vi "Launcher.vi"() -> ()   [LabVIEW 2024]
uses:
  Text/Text.lvclass
  C:/Users/burakkorkmaz/Desktop/Leveling/labview-design-patterns/Decorator Pattern/Labview/AbstractText/AbstractText.lvclass
  <vilib>/Utility/miscctls.llb/LVRectTypeDef.ctl
  BoldDecorator/BoldDecorator.lvclass
  ItalicDecorator/ItalicDecorator.lvclass
  UnderlineDecorator/UnderlineDecorator.lvclass
  AbstractText/AbstractText.lvclass
panel:
  out "Description":string
  out "Content":string
  in  "Add Underline":bool
  in  "Add Italic":bool
  in  "Add Bold":bool
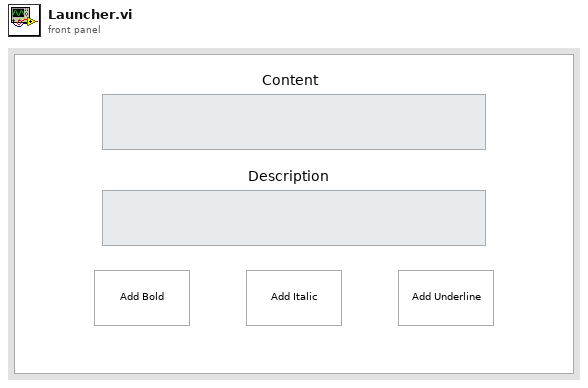
[diagram p1: front panel]
types:
  T1 = typedef "LVRectTypeDef.ctl" = cluster{"Left":i16, "Top":i16, "Right":i16, "Bottom":i16}
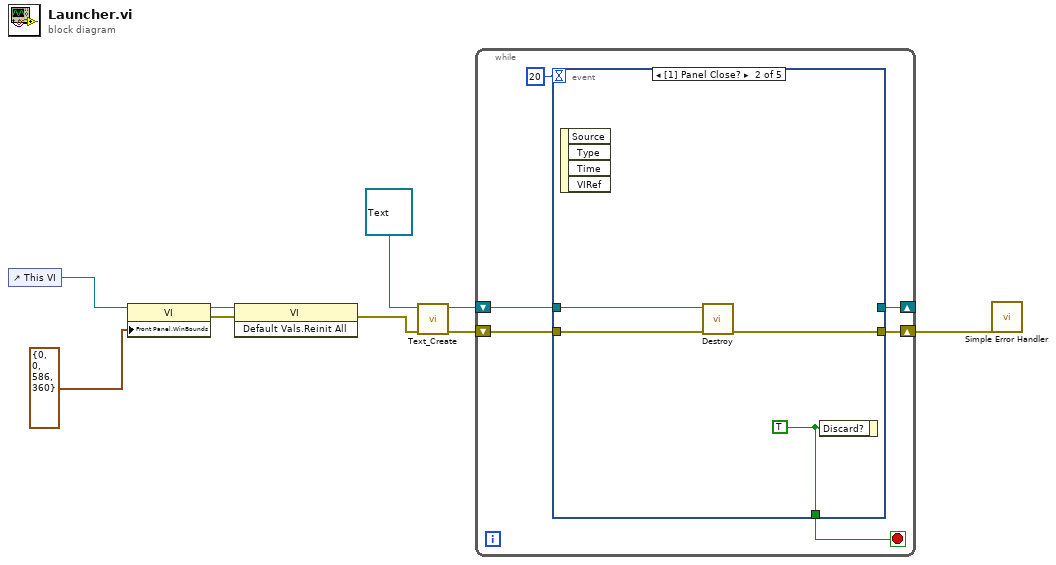
[diagram p0: block diagram]
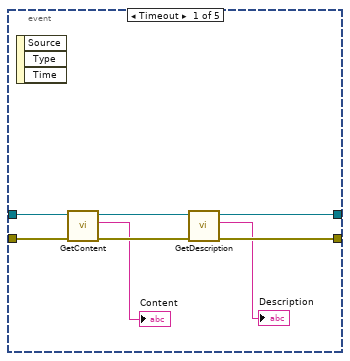
[diagram p2: hidden frame]
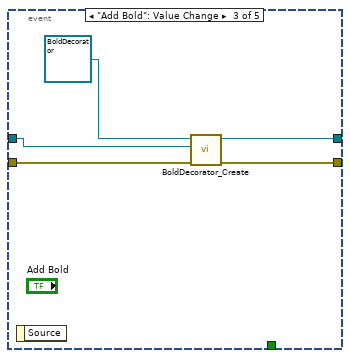
[diagram p3: hidden frame]
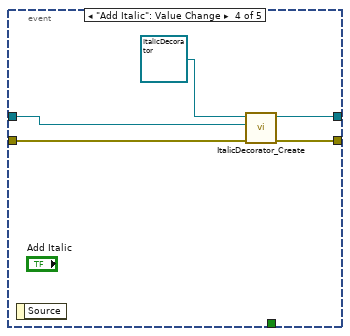
[diagram p4: hidden frame]
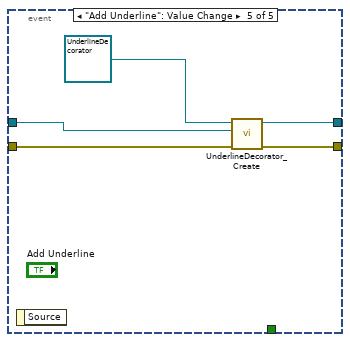
[diagram p5: hidden frame]
diagram:
  n1 = control-ref of="This VI"() -> (w9:refnum<vi>)
  n2 = property class="VI"(reference=w9, "Front Panel.WinBounds"=T1 {"Left"=0, "Top"=0, "Right"=586, "Bottom"=360} ("Front Panel Window:Window Bounds")) -> (reference out=w7:refnum<vi>, error out=w6:errorcluster)  [unwired: 1 in]
  n3 = invoke class="VI" method="Default Vals.Reinit All"(reference=w7, error in=w6) -> (error out=w5:errorcluster)  [unwired: 1 in, 2 out]
  n4 = call "Text_Create.vi"("Error In"=w5, "reference in"=refnum<class "Text.lvclass"> refnum) -> ("Error Out"=w2:errorcluster, "reference out"=w3:refnum<class "Text.lvclass">)  [unwired: 8 in]
  n5 = while {
    shift-right: [w13] -> _
    shift-left: w3 -> [w15]
    shift-right: [w12] -> w1
    shift-left: w2 -> [w14]
    stop <- w11 stop-if-true
    n6 = event shown="[1] Panel Close?" {
      selector: _ -> [_ _ _ _ _]
      dyn-events: _ -> [_ _ _ _ _]
      timeout: 20 -> [_ _ _ _ _]
      tunnel: w15 -> [w23 w24 w28 w36 w39]
      tunnel: w14 -> [w22 w26 w32 w37 w40]
      tunnel: [w19 _ w30 w34 w41] -> w13
      tunnel: [w18 w25 w31 w35 w42] -> w12
      tunnel: [_ w27 _ _ _] -> w11
      event Timeout {
        n7 = event-data() -> ()  [unwired: 1 in, 3 out]
        n8 = call-dynamic "GetContent.vi"("Error In"=w22, "reference in"=w23) -> ("Error Out"=w20:errorcluster, "Content"=→"Content":string, "reference out"=w21:refnum<class "AbstractText.lvclass">)  [unwired: 7 in]
        n9 = call-dynamic "GetDescription.vi"("Error In"=w20, "reference in"=w21) -> ("Error Out"=w18:errorcluster, "Description"=→"Description":string, "reference out"=w19:refnum<class "AbstractText.lvclass">)  [unwired: 7 in]
      }
      event Panel Close? {
        w27 = TRUE ("Discard?")
        n10 = event-data() -> ()  [unwired: 1 in, 4 out]
        n11 = call-dynamic "Destroy.vi"("Error In"=w26, "reference in"=w24) -> ("Error Out"=w25:errorcluster)  [unwired: 8 in, 1 out]
        n12 = event-data("Discard?"=w27) -> ()  [unwired: 1 in, 1 out]
      }
      event "Add Bold": Value Change {
        n13 = event-data() -> ()  [unwired: 1 in, 1 out]
        n14 = call "BoldDecorator_Create.vi"("Error In"=w32, "Text"=w28, "reference in"=refnum<class "BoldDecorator.lvclass"> refnum) -> ("Error Out"=w31:errorcluster, "reference in"=w30:refnum<class "BoldDecorator.lvclass">)  [unwired: 7 in]
      }
      event "Add Italic": Value Change {
        n15 = event-data() -> ()  [unwired: 1 in, 1 out]
        n16 = call "ItalicDecorator_Create.vi"("Error In"=w37, "Text"=w36, "reference in"=refnum<class "ItalicDecorator.lvclass"> refnum) -> ("Error Out"=w35:errorcluster, "reference in"=w34:refnum<class "ItalicDecorator.lvclass">)  [unwired: 7 in]
      }
      event "Add Underline": Value Change {
        n17 = event-data() -> ()  [unwired: 1 in, 1 out]
        n18 = call "UnderlineDecorator_Create.vi"("Error In"=w40, "AbstractText"=w39, "reference in"=refnum<class "UnderlineDecorator.lvclass"> refnum ("UnderlineDecorator")) -> ("Error Out"=w42:errorcluster, "reference in"=w41:refnum<class "UnderlineDecorator.lvclass">)  [unwired: 7 in]
      }
    }
  }
  n19 = call <vilib>:"Simple Error Handler.vi"("error in (no error)"=w1) -> ()  [unwired: 4 in, 5 out]
